vi "Error Debug.vi"(8 "error in (no error)":errorcluster, 11 "input 1":i32) -> ()   [LabVIEW 2020, in "PXI-2512 Engine.lvlib"]
uses:
  PXI-2512 Engine.lvlib
  <vilib>/Utility/SystemLogging/NI_SystemLogging.lvlib
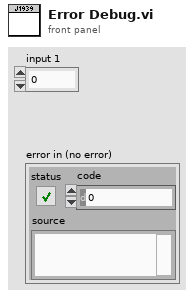
[diagram p1: front panel]
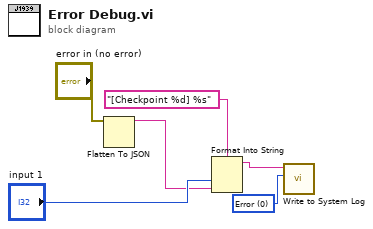
[diagram p0: block diagram]
diagram:
  w6 = 0 items=["Error", "Warning", "Informational"] ("severity")
  n1 = Flatten To JSON(anything="error in (no error)") -> (JSON string=w3:string)  [unwired: 2 in, 1 out]
  n2 = Format Into String(format string="[Checkpoint %d] %s", "input 1", w3) -> (resulting string=w5:string)  [unwired: 2 in, 1 out]
  n3 = call <vilib>:"Write to System Log.vi"("severity"=w6, "message"=w5) -> ()  [unwired: 9 in, 1 out]
